vi "Open DB.vi"(8 "error in (no error)":errorcluster, 9 "connection timeout (1)":i32=1, 10 "Connected String":string, 11 "NI_DB_API in":refnum<class "NI_DB_API.lvclass">) -> (0 "error out":errorcluster, 3 "NI_DB_API out":refnum<class "NI_DB_API.lvclass">)   [LabVIEW 2021, in "NI_DB_API.lvclass"]
uses:
  <userlib>/John_Lib/DataBase/NI_DB_API/NI_DB_API.lvclass
  <userlib>/John_Lib/DataBase/NI_DB_API/NI_DB_API.lvclass/NI_DB_API.ctl
  <vilib>/addons/database/NI_Database_API.lvlib
  <vilib>/addons/database/Connection.llb/DB Tools Open Connec (String).vi
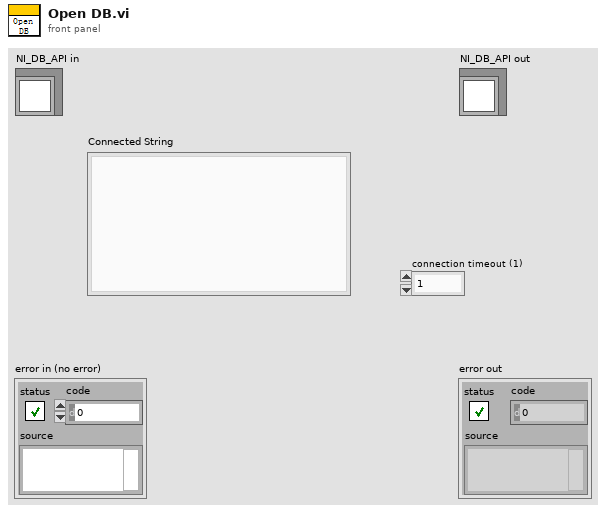
[diagram p1: front panel]
types:
  T1 = typedef "NI_Database_API.lvlib/Conn ObjectReference.ctl" = refnum<k1>
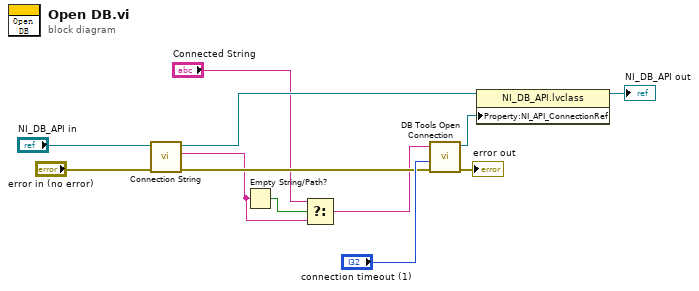
[diagram p0: block diagram]
diagram:
  n1 = call-dynamic "Connection String.vi"("error in (no error)"="error in (no error)", "DataBase_SQL in"="NI_DB_API in") -> ("error out"=w7:errorcluster, "Connected String"=w2:string, "DataBase_SQL out"=w9:refnum<class "NI_DB_API.lvclass">)  [unwired: 7 in]
  n2 = Empty String/Path?(string/path=w2) -> (empty?=w4:bool)
  n3 = Select(t="Connected String", s=w4, f=w2) -> (s? t:f=w1:string)
  n4 = call-poly <vilib>:"DB Tools Open Connection.vi"("error in (no error)"=w7, "connection timeout (15)"="connection timeout (1)", "connection information"=w1) -> ("error out"=→"error out":errorcluster, "connection reference"=w5:T1)  [unwired: 5 in]
  n5 = property class="NI_DB_API.lvclass"(reference=w9, "Property:NI_API_ConnectionRef"=w5) -> (reference out=→"NI_DB_API out":refnum<class "NI_DB_API.lvclass">)  [unwired: 1 in, 1 out]
